vi "Color Picker_Color to Component Values.vi"(7 "Select Conversion":T1=enum."HSL", 8 "Error":errorcluster, 11 "Color":u32(colorbox)) -> (0 "Error Out":errorcluster, 3 "Color Value Out":T2)   [LabVIEW 2009]
doc: "Converts color to component values"
uses:
  Color Picker Controls/Color Picker_Cluster Color Component Data Set.ctl
  Color Picker Controls/Color Picker_ENUM Color Component Select.ctl
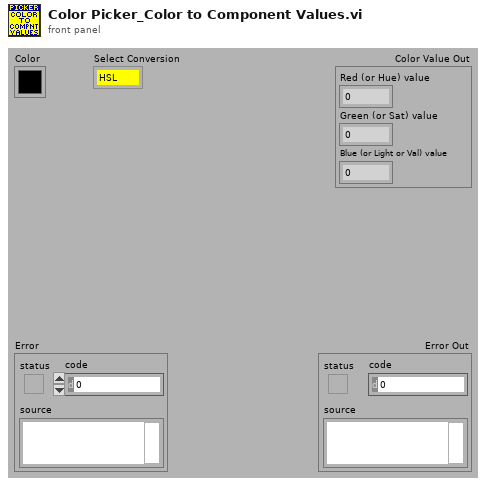
[diagram p1: front panel]
types:
  T1 = typedef "Color Picker_ENUM Color Component Select.ctl" = enum16{"RGB", "HSL"}
  T2 = typedef "Color Picker_Cluster Color Component Data Set.ctl" = cluster{"Blue (or Light or Val) value":u8, "Green (or Sat) value":u8, "Red (or Hue) value":u8}
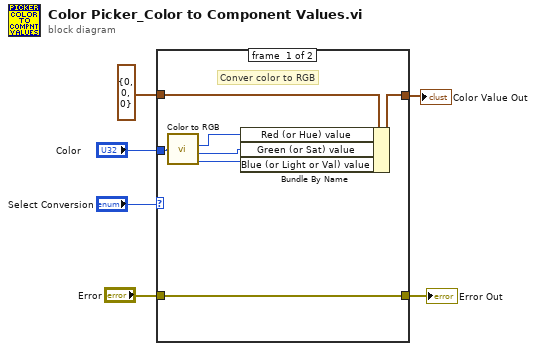
[diagram p0: block diagram]
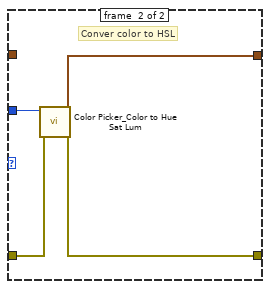
[diagram p2: hidden frame]
diagram:
  n1 = case shown="\"RGB\"" "Select Conversion" {
    tunnel: "Error" -> [w7 w15]
    tunnel: [w7 w14] -> w5
    tunnel: [w12 w17] -> w3
    tunnel: T2 {"Blue (or Light or Val) value"=0, "Green (or Sat) value"=0, "Red (or Hue) value"=0} ("Color Value") -> [w13 _]
    tunnel: "Color" -> [w8 w16]
    frame #0 {
      # "Conver color to RGB"
      n2 = call <vilib>:"Color to RGB.vi"("Color"=w8) -> ("R"=w11:u8, "G"=w10:u8, "B"=w9:u8)  [unwired: 1 out]
      n3 = Bundle By Name(cluster=w13, "Red (or Hue) value"=w11, "Green (or Sat) value"=w10, "Blue (or Light or Val) value"=w9) -> (w12:T2)
    }
    frame #1 {
      # "Conver color to HSL"
      n4 = call "Color Picker_Color to Hue Sat Lum.vi"("Error In"=w15, "Color Box"=w16) -> ("Error Out"=w14:errorcluster, "Color Value Out"=w17:T2)  [unwired: 8 in]
    }
  }
  "Color Value Out" <- w3
  "Error Out" <- w5
